vi "myRIO_BRig_RT_dataCurrent_idxDataBlockL.vi"() -> (2 "output_idxDataBlock__L":i32)   [LabVIEW 2014]
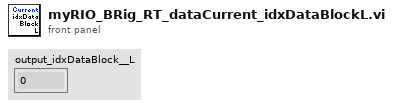
[diagram p1: front panel]
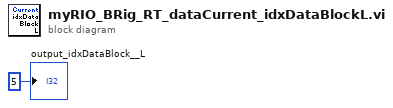
[diagram p0: block diagram]
diagram:
  "output_idxDataBlock__L" <- 5 ("output_iBlock")
